vi "rangescalc.vi"() -> ()   [LabVIEW 2015]
panel:
  in  "Min Angle":i32
  in  "Max Angle":i32
  in  "Initial Velocity":dbl
  in  "Framerate":i32
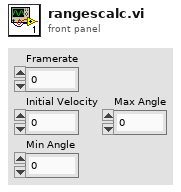
[diagram p1: front panel]
types:
  T1 = enum16{"open", "replace", "create", "open or create", "replace or create", "replace or create with confirmation"}
  T2 = cluster{"Firing Angle":dbl, "Framerate":dbl, "Initial Velocity":dbl}
  T3 = cluster{"Minimum Distance":dbl, "Ideal Distance":dbl, "Viable Distances":dbl[], "Maximum Distance":dbl}
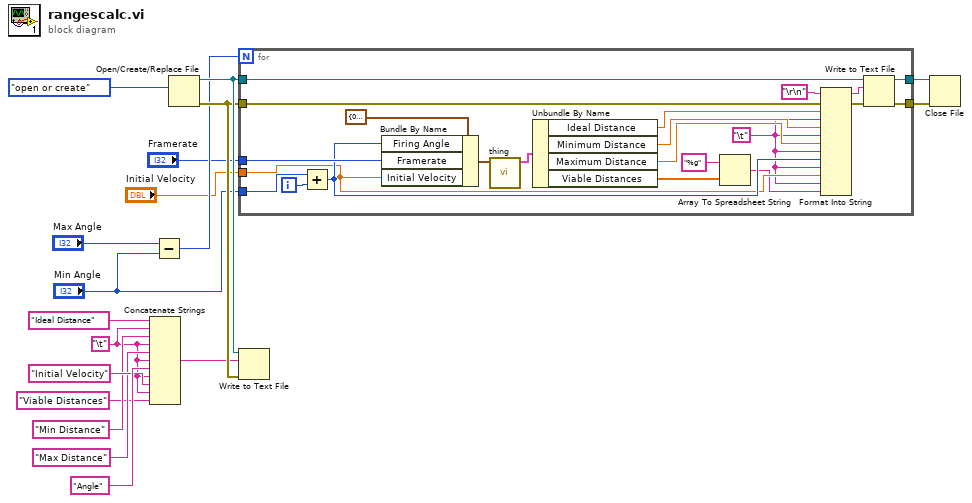
[diagram p0: block diagram]
diagram:
  w2 = "\t"
  n1 = Concatenate Strings("Ideal Distance" ("text"), w2, "Min Distance" ("text"), w2, "Max Distance" ("text"), w2, "Angle" ("string"), w2, "Initial Velocity" ("string"), w2, "Viable Distances" ("string")) -> (w11:string)
  n2 = Subtract(x="Max Angle", y="Min Angle") -> (x-y=w9:i32)
  n3 = Open/Create/Replace File(operation (0:open)=T1."open or create") -> (refnum out=w15:refnum<file>, error out=w14:errorcluster)  [unwired: 5 in, 1 out]
  n4 = for {
    N: w9 -> [_]
    tunnel: w15 -> [w40]
    tunnel: [w39] -> w17
    tunnel: [w38] -> w16
    tunnel: w14 -> [w36]
    tunnel: "Min Angle" -> [w33]
    tunnel: "Framerate" -> [w29]
    tunnel: "Initial Velocity" -> [w23]
    i -> [w32]
    w22 = "\t"
    n5 = Add(x=w33, y=w32) -> (x+y=w24:i32)
    n6 = Bundle By Name(cluster=T2 {"Firing Angle"=0.0, "Framerate"=0.0, "Initial Velocity"=0.0} ("Parameters"), "Firing Angle"=w24, "Framerate"=w29, "Initial Velocity"=w23) -> (w31:T2)
    n7 = call "thing.vi"("Parameters"=w31) -> ("Range"=w28:T3)  [unwired: 10 in]
    n8 = Unbundle By Name(w28) -> ("Ideal Distance"=w27:dbl, "Minimum Distance"=w26:dbl, "Maximum Distance"=w25:dbl, "Viable Distances"=w21:dbl[])
    n9 = Array To Spreadsheet String(array=w21, 3:"%g" ("format string")) -> (spreadsheet string=w20:string)  [unwired: 1 in]
    n10 = Format Into String(initial string="\r\n", error in=w36, w27, w22, w26, w22, w25, w22, w24, w22, w23, w22, w20) -> (resulting string=w37:string, error out=w35:errorcluster)  [unwired: 1 in]
    n11 = Write to Text File(file (use dialog)=w40, text=w37, error in=w35) -> (refnum out=w39:refnum<file>, error out=w38:errorcluster)  [unwired: 1 in, 1 out]
  }
  n12 = Write to Text File(file (use dialog)=w15, text=w11, error in=w14) -> ()  [unwired: 1 in, 3 out]
  n13 = Close File(refnum=w17, error in=w16) -> ()  [unwired: 2 out]
